vi "support_locateTaskDefFile.vi"(8 "error in (no error)":errorcluster) -> (0 "error IO":errorcluster, 3 "file path":path)   [LabVIEW 2010]
doc: "---------------------------------------------------------------\nAuthor: Dang Lam\nEmail: danglamtd@gmail.com"
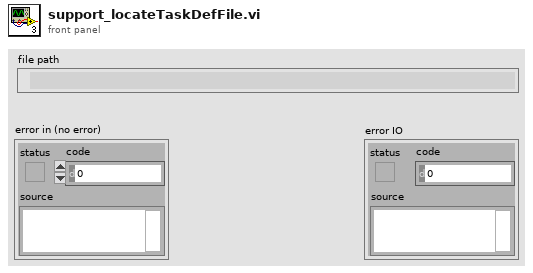
[diagram p1: front panel]
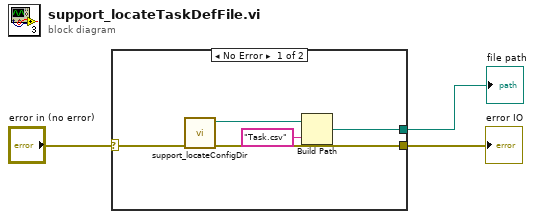
[diagram p0: block diagram]
diagram:
  n1 = case shown="No Error" "error in (no error)" {
    selector: "error in (no error)" -> [w8 w9]
    tunnel: [w7 w9] -> w2
    tunnel: [w4 _] -> w1
    frame No Error {
      n2 = call "support_locateConfigDir.vi"("error in (no error)"=w8) -> ("error IO"=w7:errorcluster, "Config path"=w6:path)  [unwired: 9 in]
      n3 = Build Path(base path=w6, name or relative path="Task.csv") -> (appended path=w4:path)
    }
    frame Error {
    }
  }
  "error IO" <- w2
  "file path" <- w1
